vi "GetSimulatedPressure.vi"(1 "Compressor On":bool) -> (0 "Simulated Pressure Transducer":dbl)   [LabVIEW 2019]
doc: "Simulates a pressure transducer by setting the pressure reading to 60 when the compressor is on and 120 when the compressor is off."
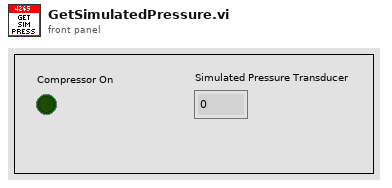
[diagram p1: front panel]
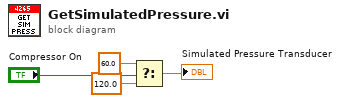
[diagram p0: block diagram]
diagram:
  n1 = Select(t=60.0, s="Compressor On", f=120.0) -> (s? t:f=→"Simulated Pressure Transducer":dbl)
